vi "MappingFunc(XYIntercept).vi"(7 "Input":dbl format="%#_13g", 10 "Cluster":T1) -> (3 "Output":dbl)   [LabVIEW 2017]
panel:
  out "XY Graph":cluster{dbl[], dbl[]}(graph)
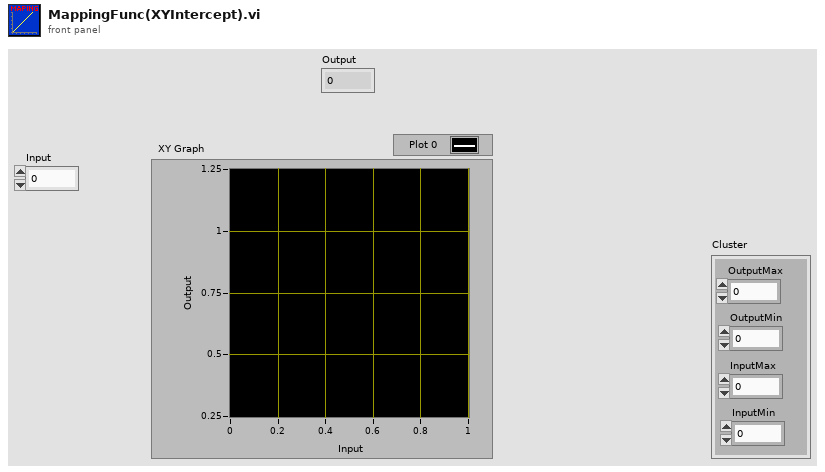
[diagram p1: front panel]
types:
  T1 = cluster{"OutputMax":dbl, "OutputMin":dbl, "InputMax":dbl, "InputMin":dbl}
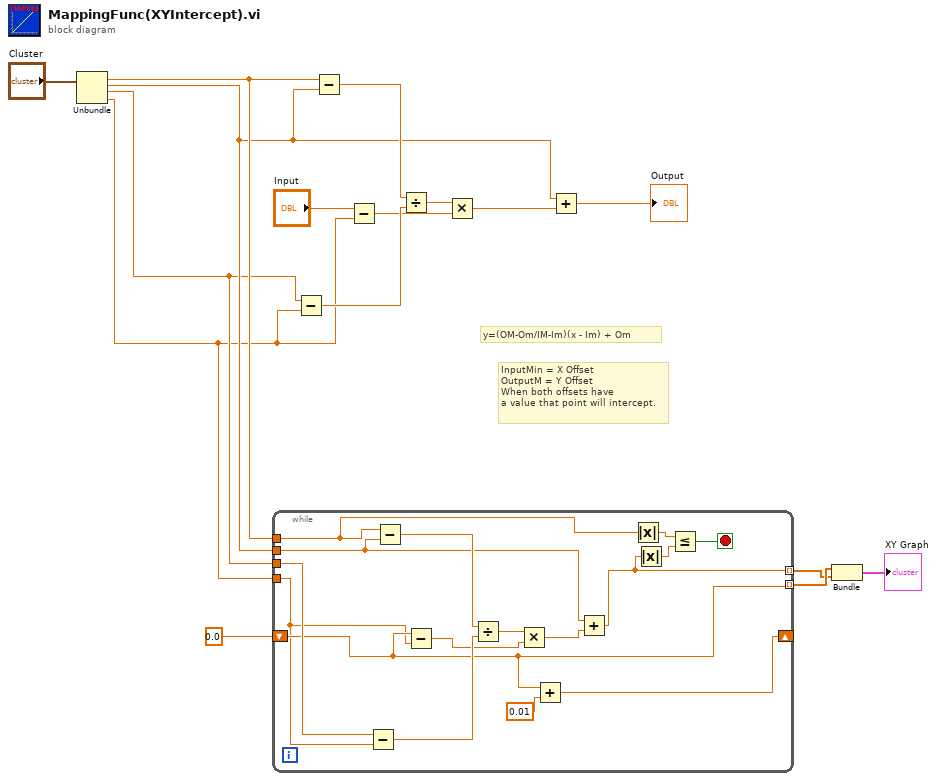
[diagram p0: block diagram]
diagram:
  # "InputMin = X Offset\nOutputM = Y Offset\nWhen both offsets have\na value that point will intercept."
  # "y=(OM-Om/IM-Im)(x - Im) + Om"
  n1 = Unbundle("Cluster") -> ("OutputMax"=w9:dbl, "OutputMin"=w7:dbl, "InputMax"=w6:dbl, "InputMin"=w5:dbl)
  n2 = while {
    tunnel: w9 -> [w20]
    tunnel: w7 -> [w17]
    tunnel: w6 -> [w29]
    tunnel: w5 -> [w24]
    shift-right: [w27] -> _
    shift-left: 0.0 -> [w26]
    tunnel: [w26] -> w3 mode=indexing
    tunnel: [w18] -> w2 mode=indexing
    stop <- w23 stop-if-true
    n3 = Subtract(x=w29, y=w24) -> (x-y=w31:dbl)
    n4 = Subtract(x=w20, y=w17) -> (x-y=w32:dbl)
    n5 = Subtract(x=w26, y=w24) -> (x-y=w25:dbl)
    n6 = Divide(x=w32, y=w31) -> (x/y=w30:dbl)
    n7 = Multiply(x=w30, y=w25) -> (x*y=w19:dbl)
    n8 = Add(x=w26, y=0.01) -> (x+y=w27:dbl)
    n9 = Add(x=w17, y=w19) -> (x+y=w18:dbl)
    n10 = Absolute Value(x=w20) -> (abs(x)=w21:dbl)
    n11 = Absolute Value(x=w18) -> (abs(x)=w22:dbl)
    n12 = Less Or Equal?(x=w21, y=w22) -> (x <= y?=w23:bool)
  }
  n13 = Subtract(x=w6, y=w5) -> (x-y=w15:dbl)
  n14 = Subtract(x=w9, y=w7) -> (x-y=w16:dbl)
  n15 = Subtract(x="Input", y=w5) -> (x-y=w12:dbl)
  n16 = Divide(x=w16, y=w15) -> (x/y=w14:dbl)
  n17 = Multiply(x=w14, y=w12) -> (x*y=w10:dbl)
  n18 = Add(x=w7, y=w10) -> (x+y=→"Output":dbl)
  n19 = Bundle(w3, w2) -> (→"XY Graph":cluster{dbl[], dbl[]})  [unwired: 1 in]
